vi "Circular Buffer Array-8.6.vi"(9 "Array Size":dbl=10.0, 11 "new element/subarray 2":dbl) -> (3 "Circular Array":dbl[](array[numeric]))   [LabVIEW 2014]
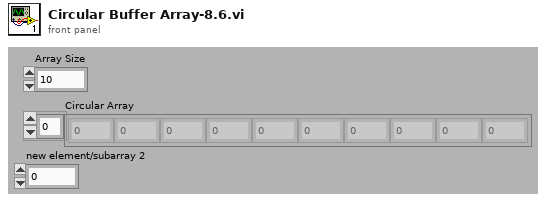
[diagram p1: front panel]
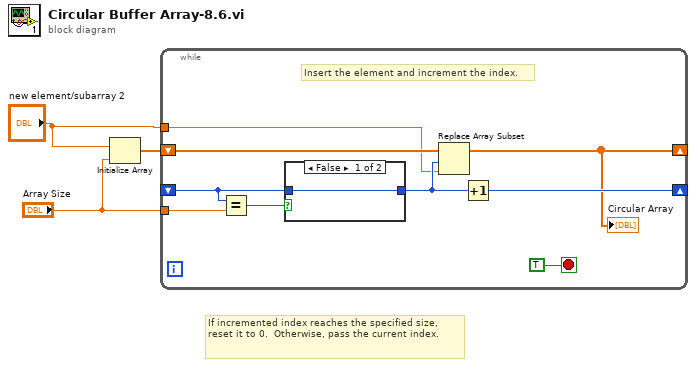
[diagram p0: block diagram]
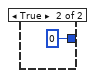
[diagram p2: hidden frame]
diagram:
  # "If incremented index reaches the specified size, reset it to 0.  Otherwise, pass the current index."
  n1 = Initialize Array("new element/subarray 2", "Array Size") -> (w3:dbl[])
  n2 = while {
    shift-right: [w9] -> _
    shift-left: _ -> [w11]
    shift-right: [w7] -> _
    shift-left: w3 -> [w5]
    tunnel: "Array Size" -> [w8]
    tunnel: "new element/subarray 2" -> [w4]
    stop <- TRUE stop-if-true
    # "Insert the element and increment the index."
    n3 = Equal?(x=w11, y=w8) -> (x = y?=w12:bool)
    n4 = case shown="False" w12 {
      tunnel: w11 -> [w13 _]
      tunnel: [w13 0] -> w10
      frame False {
      }
      frame True {
      }
    }
    n5 = Replace Array Subset "Replace Array Subset"(array=w5, new element=w4, index=w10) -> (w7:dbl[])
    "Circular Array" <- w7
    n6 = Increment(x=w10) -> (x+1=w9:i32)
  }
